vi "ConfigDlg.vi"(8 "error in (no error)":errorcluster, 11 "IviFgen in":refnum<class "IviFgen.lvclass">) -> (0 "error out":errorcluster, 2 "Changed":bool, 3 "IviFgen out":refnum<class "IviFgen.lvclass">)   [LabVIEW 2014, in "FgenPlugins.lvlib" / "IviFgen.lvclass"]
uses:
  IviFgen.lvclass
  TypeDefs/Channel.ctl
  TypeDefs/clTriggers.ctl
  TypeDefs/Trigger.ctl
  TypeDefs/TriggerType.ctl
  FgenPluginBaseClass/FgenPluginsBase.lvclass/FgenPluginsBase.ctl
  <userlib>/NIST/BaseClasses/BasePlugin_class/BasePlugin.lvclass/BasePlugin.ctl
  <userlib>/NIST/BaseClasses/BasePlugin_class/Accessors/Read PluginIniFilePath.vi
  FgenPluginBaseClass/Accessors/Write reference clock source (Internal).vi
  FgenPluginBaseClass/Accessors/Write Triggers.vi
  FgenPluginBaseClass/Accessors/Write Channels.vi
  FgenPluginBaseClass/Accessors/Read FunctionClass.vi
  FgenPluginBaseClass/Accessors/Write FunctionClass.vi
  FgenPluginBaseClass/Accessors/Read Channels.vi
  FgenPluginBaseClass/Accessors/Read reference clock source (Internal).vi
  FgenPluginBaseClass/Read Triggers.vi
  MemberClasses/FunctionBaseClass/FunctionBase.lvclass
  <vilib>/Utility/config.llb/NI_LVConfig.lvlib
  FgenPlugins.lvlib
panel:
  in  "Triggers":T1
  in  "reference clock source (Internal)":i32 caption="Ref Clk Src"
  in  "Channels":cluster{"Count":u16, "Channel":T4[]}
  in  "btnDone":bool
  in  "btnCancel":bool
  in  "btnFuncConfig":bool
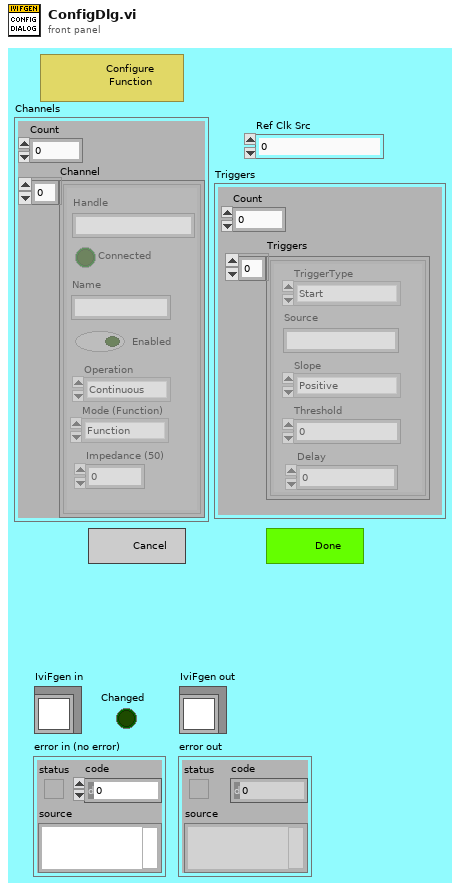
[diagram p1: front panel]
types:
  T1 = typedef "FgenPlugins.lvlib/clTriggers.ctl" = cluster{"Count":i32, "Triggers":T2[]}
  T2 = typedef "FgenPlugins.lvlib/Trigger.ctl" = cluster{"Source":string, "Slope":enum16{"Positive", "Negative", "Either"}, "Threshold":dbl, "Delay":dbl, "TriggerType":T3}
  T3 = typedef "FgenPlugins.lvlib/TriggerType.ctl" = enum16{"None", "Start", "Stop", "Hold", "Resume", "Advance"}
  T4 = typedef "FgenPlugins.lvlib/Channel.ctl" = cluster{"Name":string, "Enabled":bool, "Operation":enum16{"Continuous", "Burst"}, "Impedance (50)":dbl, "Handle":string, "Connected":bool, "Mode (Function)":enum16{"Function", "Arbitrary", "Sequence"}}
  T5 = typedef "NI_LVConfig.lvlib/Config Data RefNum.ctl" = refnum<k1>
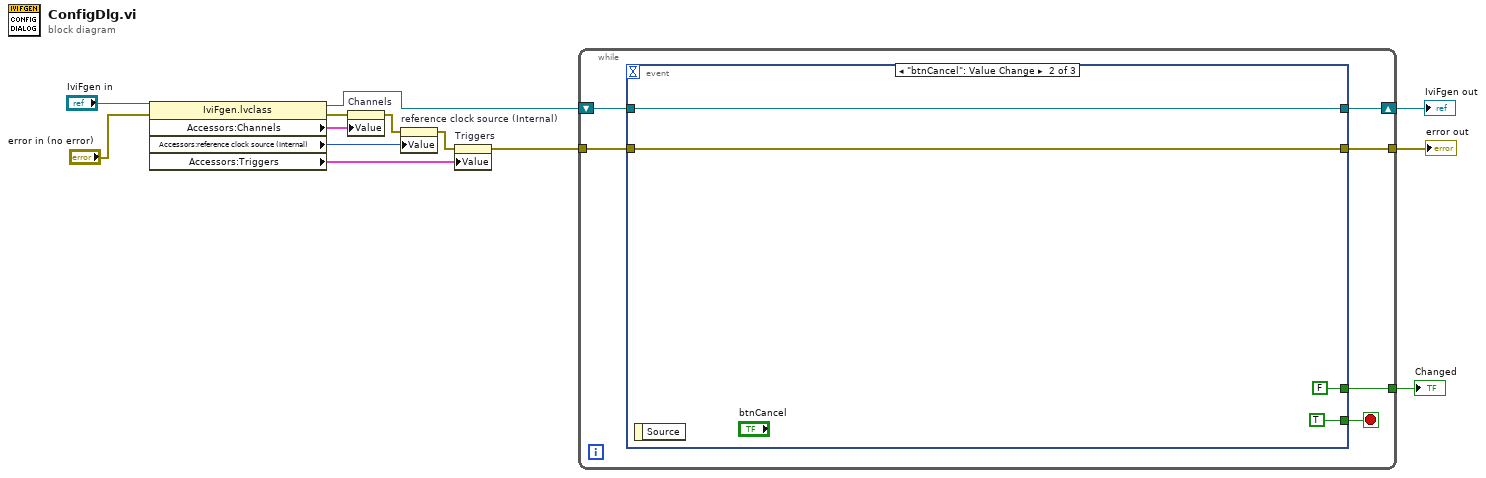
[diagram p0: block diagram]
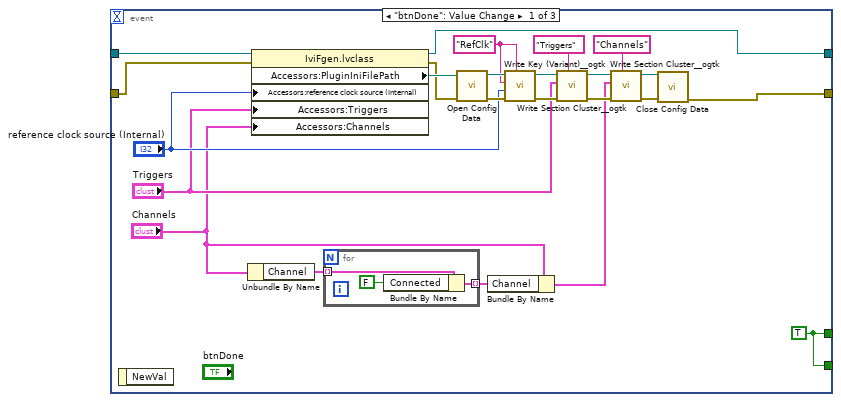
[diagram p2: hidden frame]
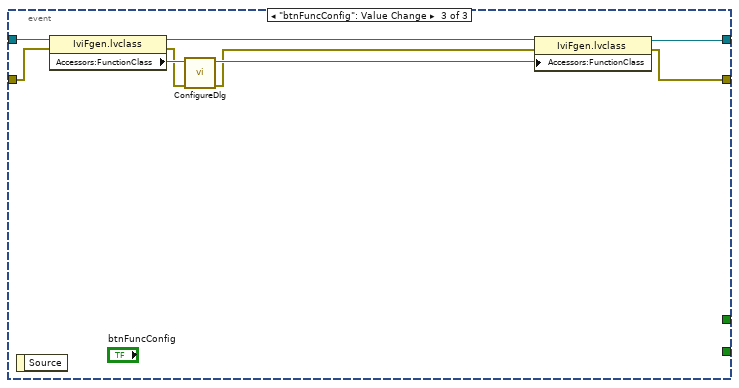
[diagram p3: hidden frame]
diagram:
  n1 = property class="IviFgen.lvclass"(reference="IviFgen in", error in="error in (no error)") -> (reference out=w5:refnum<class "IviFgen.lvclass">, error out=w11:errorcluster, "Accessors:Channels"=w10:cluster{"Count":u16, "Channel":T4[]}, "Accessors:reference clock source (Internal)"=w9:i32, "Accessors:Triggers"=w7:T1)
  n2 = property on="Channels" class="Clust (strict)"(error in=w11, "Value"=w10) -> (error out=w8:errorcluster)  [unwired: 1 in, 1 out]
  n3 = property on="reference clock source (Internal)" class="DigNum (strict)"(error in=w8, "Value"=w9) -> (error out=w6:errorcluster)  [unwired: 1 in, 1 out]
  n4 = property on="Triggers" class="Clust (strict)"(error in=w6, "Value"=w7) -> (error out=w3:errorcluster)  [unwired: 1 in, 1 out]
  n5 = while {
    shift-right: [w15] -> w2
    shift-left: w5 -> [w17]
    tunnel: [w18] -> w4
    tunnel: w3 -> [w16]
    tunnel: [w14] -> w1
    stop <- w19 stop-if-true
    n6 = event shown="[1] \"btnCancel\": Value Change" {
      selector: _ -> [_ _ _]
      dyn-events: _ -> [_ _ _]
      timeout: _ -> [_ _ _]
      tunnel: [w43 TRUE _] -> w19
      tunnel: [w43 FALSE _] -> w18
      tunnel: w17 -> [w42 w50 w59]
      tunnel: [w26 w49 w51] -> w14
      tunnel: w16 -> [w25 w49 w58]
      tunnel: [w20 w50 w52] -> w15
      event "btnDone": Value Change {
        w37 = "RefClk" ("section")
        w43 = TRUE
        n7 = event-data() -> ()  [unwired: 1 in, 1 out]
        n8 = Unbundle By Name("Channels") -> ("Channel"=w24:T4[])
        n9 = property class="IviFgen.lvclass"(reference=w42, error in=w25, "Accessors:reference clock source (Internal)"="reference clock source (Internal)", "Accessors:Triggers"="Triggers", "Accessors:Channels"="Channels") -> (reference out=w20:refnum<class "IviFgen.lvclass">, error out=w40:errorcluster, "Accessors:PluginIniFilePath"=w41:path)
        n10 = for {
          tunnel: w24 -> [w46] mode=indexing
          tunnel: [w44] -> w23 mode=indexing
          n11 = Bundle By Name(cluster=w46, "Connected"=FALSE) -> (w44:T4)
        }
        n12 = call <vilib>:"Open Config Data.vi"("error in (no error)"=w40, "configuration file path"=w41) -> ("error out"=w39:errorcluster, "refnum"=w38:T5)  [unwired: 7 in, 1 out]
        n13 = Bundle By Name(cluster="Channels", "Channel"=w23) -> (w22:cluster{"Count":u16, "Channel":T4[]})
        n14 = call <userlib>:"Write Key (Variant)__ogtk.vi"("section"=w37, "error in (no error)"=w39, "key-value"="reference clock source (Internal)", "key (optional)"=w37, "refnum"=w38) -> ("error out"=w35:errorcluster, "refnum out"=w34:T5)  [unwired: 5 in]
        n15 = call <userlib>:"Write Section Cluster__ogtk.vi"("section (optional)"="Triggers", "error in (no error)"=w35, "Section Formatted Cluster"="Triggers", "refnum"=w34) -> ("error out"=w31:errorcluster, "dup refnum"=w30:T5)  [unwired: 6 in]
        n16 = call <userlib>:"Write Section Cluster__ogtk.vi"("section (optional)"="Channels", "error in (no error)"=w31, "Section Formatted Cluster"=w22, "refnum"=w30) -> ("error out"=w28:errorcluster, "dup refnum"=w27:T5)  [unwired: 6 in]
        n17 = call <vilib>:"Close Config Data.vi"("error in (no error)"=w28, "refnum"=w27) -> ("error out"=w26:errorcluster)  [unwired: 8 in, 1 out]
      }
      event "btnCancel": Value Change {
        n18 = event-data() -> ()  [unwired: 1 in, 1 out]
      }
      event "btnFuncConfig": Value Change {
        n19 = event-data() -> ()  [unwired: 1 in, 1 out]
        n20 = property class="IviFgen.lvclass"(reference=w59, error in=w58) -> (reference out=w55:refnum<class "IviFgen.lvclass">, error out=w56:errorcluster, "Accessors:FunctionClass"=w57:refnum<class "FunctionBase.lvclass">)
        n21 = call-dynamic "ConfigureDlg.vi"("error in (no error)"=w56, "FunctionBase in"=w57) -> ("error out"=w53:errorcluster, "FunctionBase out"=w54:refnum<class "FunctionBase.lvclass">)  [unwired: 7 in, 1 out]
        n22 = property class="IviFgen.lvclass"(reference=w55, error in=w53, "Accessors:FunctionClass"=w54) -> (reference out=w52:refnum<class "IviFgen.lvclass">, error out=w51:errorcluster)
      }
    }
  }
  "error out" <- w1
  "IviFgen out" <- w2
  "Changed" <- w4
